vi "Open Bundle.vi"(8 "error in (no error)":errorcluster, 11 "Bundle Builder in":refnum<class "Bundle Builder.lvclass">) -> (0 "error out":errorcluster, 1 "Custom Actions File Names":string[](array[string]), 2 "Product List File Names":string[](array[string]), 3 "Bundle Builder out":refnum<class "Bundle Builder.lvclass">, 4 "Bundle Filename":string)   [LabVIEW 2020, in "Bundle Builder.lvclass"]
uses:
  Bundle Builder.lvclass
  Bundle Builder.lvclass/Bundle Builder.ctl
  C:/Users/chihong/Documents/Repos/StsCustomBundleBuilder/StsCustomBundleBuilder/StsCustomBundleBuilderLib/StsCustomBundleBuilderLib.dll
  StsCustomBundleBuilderLib/StsCustomBundleBuilderLib.dll
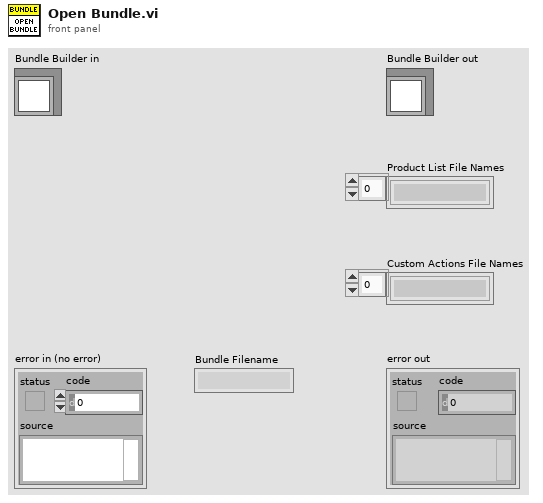
[diagram p1: front panel]
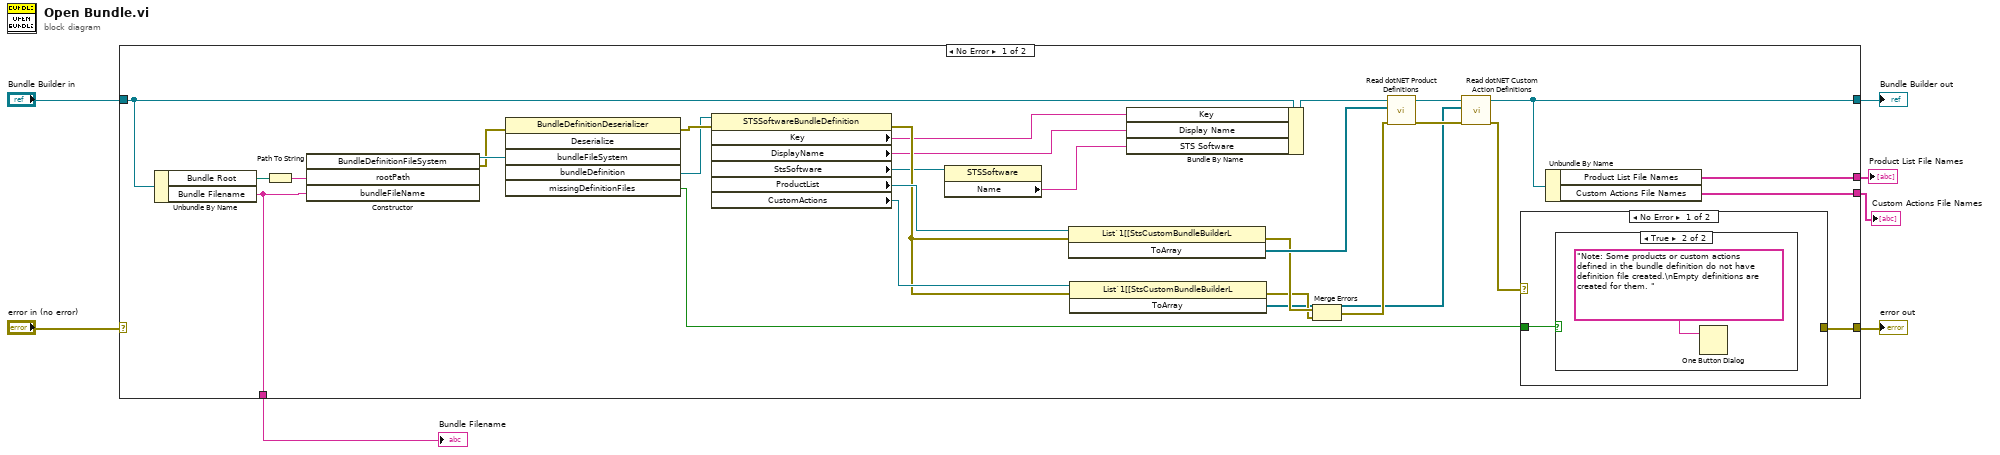
[diagram p0: block diagram]
diagram:
  n1 = case shown="No Error" "error in (no error)" {
    selector: "error in (no error)" -> [_ w41]
    tunnel: [w8 w41] -> w6
    tunnel: [w19 w40] -> w4
    tunnel: "Bundle Builder in" -> [w36 w40]
    tunnel: [w27 _] -> w3
    tunnel: [w18 _] -> w2
    tunnel: [w17 _] -> w1
    frame No Error {
      n2 = Unbundle By Name(w36) -> ("Bundle Root"=w35:path, "Bundle Filename"=w27:string)
      n3 = Path To String(path=w35) -> (string=w34:string)
      n4 = constructor class="BundleDefinitionFileSystem"("rootPath"=w34, "bundleFileName"=w27) -> (reference out=w33:refnum<k24>, error out=w32:errorcluster)  [unwired: 3 in, 3 out]
      n5 = invoke class="BundleDefinitionDeserializer" method="Deserialize"(error in=w32, "bundleFileSystem"=w33) -> (error out=w28:errorcluster, "bundleDefinition"=w16:refnum<k24>, "missingDefinitionFiles"=w9:bool)  [unwired: 4 in, 3 out]
      n6 = property class="STSSoftwareBundleDefinition"(reference=w16, error in=w28) -> (error out=w29:errorcluster, "Key"=w11:string, "DisplayName"=w12:string, "StsSoftware"=w14:refnum<k24>, "ProductList"=w31:refnum<k24>, "CustomActions"=w30:refnum<k24>)  [unwired: 1 out]
      n7 = property class="STSSoftware"(reference=w14) -> ("Name"=w13:string)  [unwired: 1 in, 2 out]
      n8 = invoke class="List`1[[StsCustomBundleBuilderL" method="ToArray"(reference=w31, error in=w29) -> (error out=w24:errorcluster, "ToArray"=w25:refnum<k24>[])  [unwired: 1 in, 1 out]
      n9 = invoke class="List`1[[StsCustomBundleBuilderL" method="ToArray"(reference=w30, error in=w29) -> (error out=w21:errorcluster, "ToArray"=w20:refnum<k24>[])  [unwired: 1 in, 1 out]
      n10 = Bundle By Name(cluster=w36, "Key"=w11, "Display Name"=w12, "STS Software"=w13) -> (w15:refnum<class "Bundle Builder.lvclass">)
      n11 = Merge Errors(w24, w21) -> (w22:errorcluster)
      n12 = call "Read dotNET Product Definitions.vi"("error in (no error)"=w22, "Product Definitions"=w25, "Bundle Builder in"=w15) -> ("error out"=w23:errorcluster, "Bundle Builder out"=w26:refnum<class "Bundle Builder.lvclass">)  [unwired: 7 in]
      n13 = call "Read dotNET Custom Action Definitions.vi"("error in (no error)"=w23, "Custom Action Definitions"=w20, "Bundle Builder in"=w26) -> ("error out"=w10:errorcluster, "Bundle Builder out"=w19:refnum<class "Bundle Builder.lvclass">)  [unwired: 7 in]
      n14 = case shown="No Error" w10 {
        selector: w10 -> [_ w39]
        tunnel: w9 -> [w37 _]
        tunnel: [_ w39] -> w8
        frame No Error {
          n15 = case shown="True" w37 {
            frame False {
            }
            frame True {
              n16 = One Button Dialog(message="Note: Some products or custom actions defined in the bundle definition do not have definition file created.\nEmpty definitions are created for them. ") -> ()  [unwired: 1 in, 1 out]
            }
          }
        }
        frame Error {
        }
      }
      n17 = Unbundle By Name(w19) -> ("Product List File Names"=w18:string[], "Custom Actions File Names"=w17:string[])
    }
    frame Error {
    }
  }
  "error out" <- w6
  "Bundle Builder out" <- w4
  "Product List File Names" <- w2
  "Custom Actions File Names" <- w1
  "Bundle Filename" <- w3
